vi "Print Error.vi"(8 "error in (no error)":errorcluster) -> ()   [LabVIEW 2012, in "Shared Variable Custom Device.lvlib"]
uses:
  Shared Variable Custom Device.lvlib
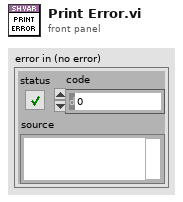
[diagram p1: front panel]
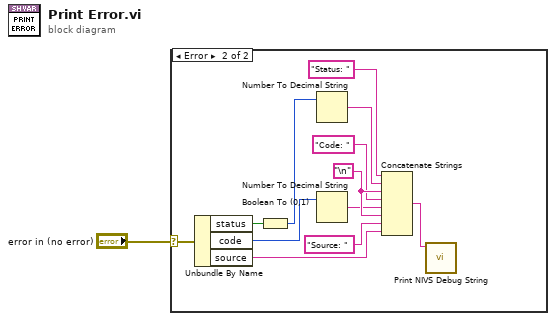
[diagram p0: block diagram]
diagram:
  n1 = case shown="Error" "error in (no error)" {
    selector: "error in (no error)" -> [_ w2]
    frame No Error {
    }
    frame Error {
      w11 = "\n"
      n2 = Unbundle By Name(w2) -> ("status"=w4:bool, "code"=w9:i32, "source"=w13:string)
      n3 = Boolean To (0,1)(Boolean=w4) -> (0, 1=w5:i16)
      n4 = Number To Decimal String(number=w5) -> (decimal integer string=w6:string)  [unwired: 1 in]
      n5 = Number To Decimal String(number=w9) -> (decimal integer string=w10:string)  [unwired: 1 in]
      n6 = Concatenate Strings("Status: " ("string"), w6, w11, "Code: " ("string"), w10, w11, "Source: " ("string"), w13) -> (w3:string)
      n7 = call "Print NIVS Debug String.vi"("Debug String"=w3) -> ()  [unwired: 9 in, 1 out]
    }
  }
